vi "move_to_next.vi"(6 "CURRENT VALVE":u32, 8 "error in (no error)":errorcluster, 9 "# REACTORS":u32, 10 "REACTORS TO USE":u32[](array[numeric]), 11 "VISA Refnum in":refnum<visa-resource-name>) -> (0 "error out":errorcluster, 3 "New Position":u32)   [LabVIEW 2013]
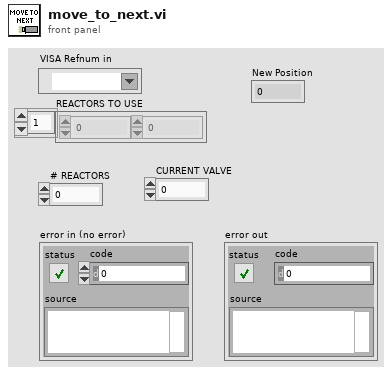
[diagram p1: front panel]
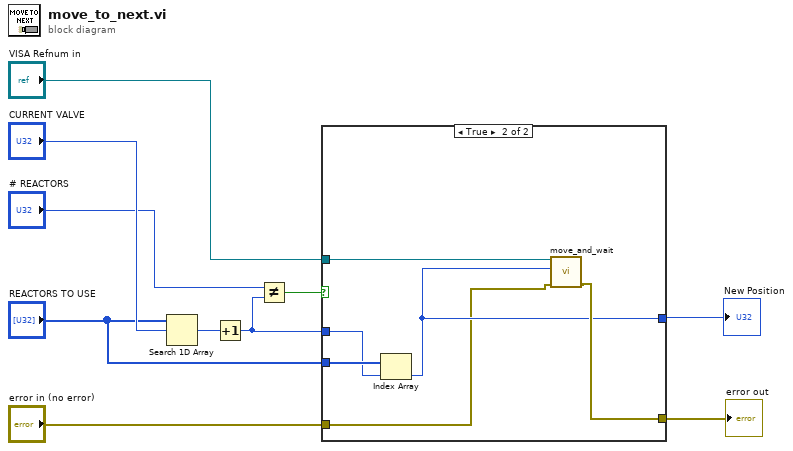
[diagram p0: block diagram]
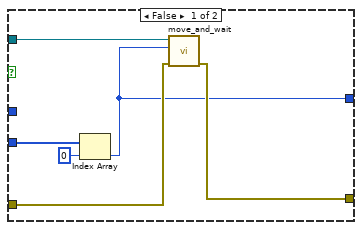
[diagram p2: hidden frame]
diagram:
  n1 = Search 1D Array(1D array="REACTORS TO USE", element="CURRENT VALVE") -> (index of element=w4:i32)  [unwired: 1 in]
  n2 = Increment(x=w4) -> (x+1=w2:i32)
  n3 = Not Equal?(x="# REACTORS", y=w2) -> (x != y?=w9:bool)
  n4 = case shown="True" w9 {
    tunnel: "REACTORS TO USE" -> [w15 w22]
    tunnel: "VISA Refnum in" -> [w16 w19]
    tunnel: "error in (no error)" -> [w13 w17]
    tunnel: [w12 w20] -> w5
    tunnel: w2 -> [_ w21]
    tunnel: [w11 w18] -> w1
    frame False {
      n5 = Index Array(array=w15, index=0) -> (element=w11:u32)
      n6 = call "move_and_wait.vi"("Error IN"=w13, "MOVE TO POSITION"=w11, "VISA Resource IN"=w16) -> ("Error OUT"=w12:errorcluster)  [unwired: 6 in, 2 out]
    }
    frame True {
      n7 = Index Array(array=w22, index=w21) -> (element=w18:u32)
      n8 = call "move_and_wait.vi"("Error IN"=w17, "MOVE TO POSITION"=w18, "VISA Resource IN"=w19) -> ("Error OUT"=w20:errorcluster)  [unwired: 6 in, 2 out]
    }
  }
  "error out" <- w5
  "New Position" <- w1
